vi "tank drive recorder.vi"(0 "leftSpeed":dbl, 1 "rightSpeed":dbl, 3 "motorController":string, 5 "stop":bool, 6 "driveMotors":string, 7 "leftMotor":string, 9 "rightMotor":string) -> (14 "distanceLeft":dbl, 15 "distanceRight":dbl)   [LabVIEW 2019, in "Encoder Recorder.lvlib"]
uses:
  Encoder Recorder.lvlib
  <vilib>/Rock Robotics/WPI/Utilities/WPI_GetSetVariantRefNum.vi
  <vilib>/Rock Robotics/WPI/ThirdParty/Phoenix-LabVIEW/Motor Controller/Get/CTRE_Phoenix_MotorController_GetSelectedSensorData.vi
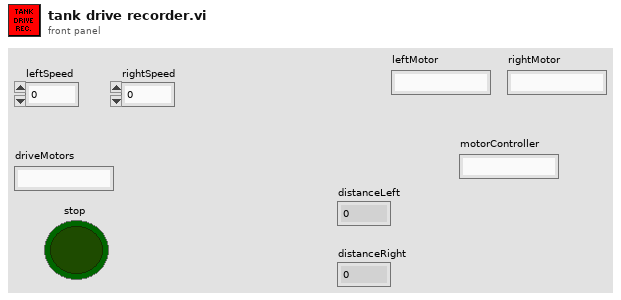
[diagram p1: front panel]
types:
  T1 = typedef "WPI_MotorControlDeviceRef.ctl" = cluster{"DeviceStatus":errorcluster, "Type":T2, "PWM":cluster{"PWM Channel":T3, "DeadBand":T4}, "CAN":cluster{"Device Number":u8, "SetOutput VI Ref":variant, "GetOutput VI Ref":variant, "Enable VI Ref":variant, "Disable VI Ref":variant, "Data":variant}, "Invert":bool, "DIO PWM":cluster{"PWM \"Enable\" Channel":T3, "DIOChannel":T5, "PWM Rate":dbl}}
  T2 = typedef "WPI_MotorControlType.ctl" = enum16{"PWM", "CAN", "DIO PWM"}
  T3 = typedef "FPGA_DIOPWMChannel.ctl" = enum8{"PWM 0", "PWM 1", "PWM 2", "PWM 3", "PWM 4", "PWM 5", "PWM 6", "PWM 7", "PWM 8", "PWM 9", "PWM MXP 0", "PWM MXP 1", "PWM MXP 2", "PWM MXP 3", "PWM MXP 4", "PWM MXP 5", "PWM MXP 6", "PWM MXP 7", "PWM MXP 8", "PWM MXP 9", "Invalid"}
  T4 = typedef "WPI_PWMDeadband.ctl" = cluster{"Name":string, "maxPositivePwm":i32, "minPositivePwm":i32, "centerPwm":i32, "maxNegativePwm":i32, "minNegativePwm":i32, "angularRange":u16}
  T5 = typedef "FPGA_DIOChannel.ctl" = enum8{"DIO 0", "DIO 1", "DIO 2", "DIO 3", "DIO 4", "DIO 5", "DIO 6", "DIO 7", "DIO 8", "DIO 9", "DIO MXP 0", "DIO MXP 1", "DIO MXP 2", "DIO MXP 3", "DIO MXP 4", "DIO MXP 5", "DIO MXP 6", "DIO MXP 7", "DIO MXP 8", "DIO MXP 9", "DIO MXP 10", "DIO MXP 11", "DIO MXP 12", "DIO MXP 13", "DIO MXP 14", "DIO MXP 15", "SPI Port CS1", "SPI Port CS2", "SPI Port CS3", "SPI Port MISO", "SPI Port MOSI", "Invalid"}
  T6 = typedef "WPI_RobotDriveDevRef.ctl" = cluster{"DevStatus":errorcluster, "Motors[]":T1[], "Square Inputs":bool, "Max Output":dbl}
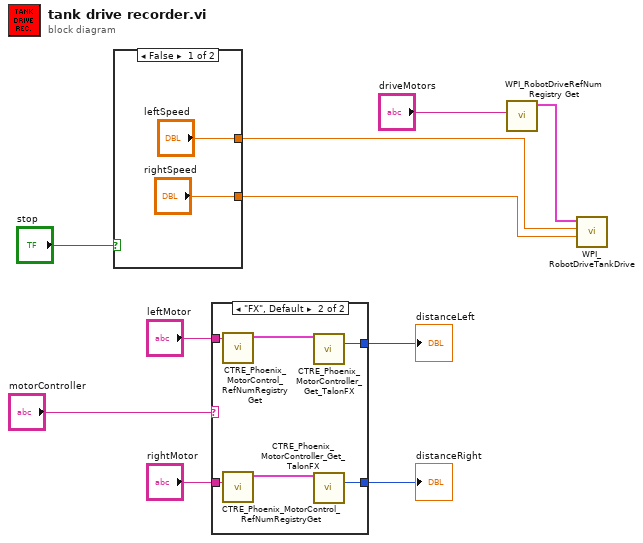
[diagram p0: block diagram]
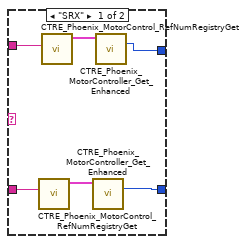
[diagram p2: hidden frame]
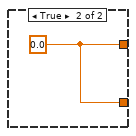
[diagram p3: hidden frame]
diagram:
  n1 = case shown="False" "stop" {
    tunnel: ["leftSpeed" w13] -> w7
    tunnel: ["rightSpeed" w13] -> w6
    frame False {
    }
    frame True {
      w13 = 0.0 ("leftSpeed")
    }
  }
  n2 = case shown="\"FX\", Default" "motorController" {
    tunnel: "leftMotor" -> [w19 w25]
    tunnel: [w18 w23] -> w4
    tunnel: [w16 w21] -> w3
    tunnel: "rightMotor" -> [w15 w20]
    frame "SRX" {
      n3 = call <vilib>:"CTRE_Phoenix_MotorControl_RefNumRegistryGet.vi"("refnum name"=w15) -> ("PhoenixMotorControlDevRef"=w14:T1)  [unwired: 9 in, 1 out]
      n4 = call <vilib>:"CTRE_Phoenix_MotorControl_RefNumRegistryGet.vi"("refnum name"=w19) -> ("PhoenixMotorControlDevRef"=w17:T1)  [unwired: 9 in, 1 out]
      n5 = call-poly <vilib>:"CTRE_Phoenix_MotorController_Get_Enhanced.vi"("PhoenixMotorControlDevRef"=w14) -> ("Position (Raw Sensor Units)"=w16:i32)  [unwired: 11 in, 3 out]
      n6 = call-poly <vilib>:"CTRE_Phoenix_MotorController_Get_Enhanced.vi"("PhoenixMotorControlDevRef"=w17) -> ("Position (Raw Sensor Units)"=w18:i32)  [unwired: 11 in, 3 out]
    }
    frame "FX", Default {
      n7 = call <vilib>:"CTRE_Phoenix_MotorControl_RefNumRegistryGet.vi"("refnum name"=w25) -> ("PhoenixMotorControlDevRef"=w24:T1)  [unwired: 9 in, 1 out]
      n8 = call <vilib>:"CTRE_Phoenix_MotorControl_RefNumRegistryGet.vi"("refnum name"=w20) -> ("PhoenixMotorControlDevRef"=w22:T1)  [unwired: 9 in, 1 out]
      n9 = call-poly <vilib>:"CTRE_Phoenix_MotorController_Get_TalonFX.vi"("PhoenixMotorControlDevRef"=w24) -> ("Position (Raw Sensor Units)"=w23:i32)  [unwired: 11 in, 3 out]
      n10 = call-poly <vilib>:"CTRE_Phoenix_MotorController_Get_TalonFX.vi"("PhoenixMotorControlDevRef"=w22) -> ("Position (Raw Sensor Units)"=w21:i32)  [unwired: 11 in, 3 out]
    }
  }
  "distanceLeft" <- w4
  "distanceRight" <- w3
  n11 = call <vilib>:"WPI_RobotDriveRefNum Registry Get.vi"("refnum name"="driveMotors") -> ("RobotDriveDevRef"=w8:T6)  [unwired: 9 in, 1 out]
  n12 = call <vilib>:"WPI_RobotDriveTankDrive.vi"("Right axis value"=w6, "Left axis value"=w7, "RobotDriveDevRef"=w8) -> ()  [unwired: 6 in, 3 out]
